vi "Global.vi"() -> ()   [LabVIEW 2010]
panel:
  in  "Edit?":bool
  in  "Index":i32
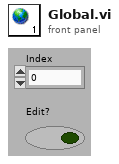
[diagram p1: front panel]
diagram:
